vi "SetSequenceNegativeTransitionRegister.vi"(8 "Error In":errorcluster, 10 "Sequence Negative Transition Register":bool[](array[boolean]), 11 "Keithley 7001 In":refnum<visa-resource-name>) -> (0 "Error Out":errorcluster, 3 "Keithley 7001 Out":refnum<visa-resource-name>)   [LabVIEW 2012, in "Keithley-7001.lvlib"]
uses:
  Keithley-7001.lvlib
panel:
  # "Lay1"
  # "Lay2"
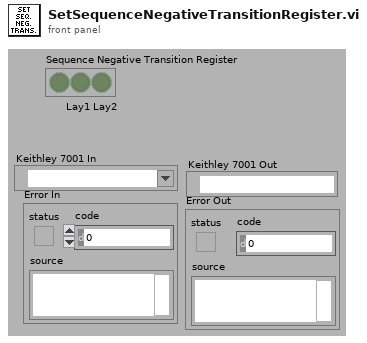
[diagram p1: front panel]
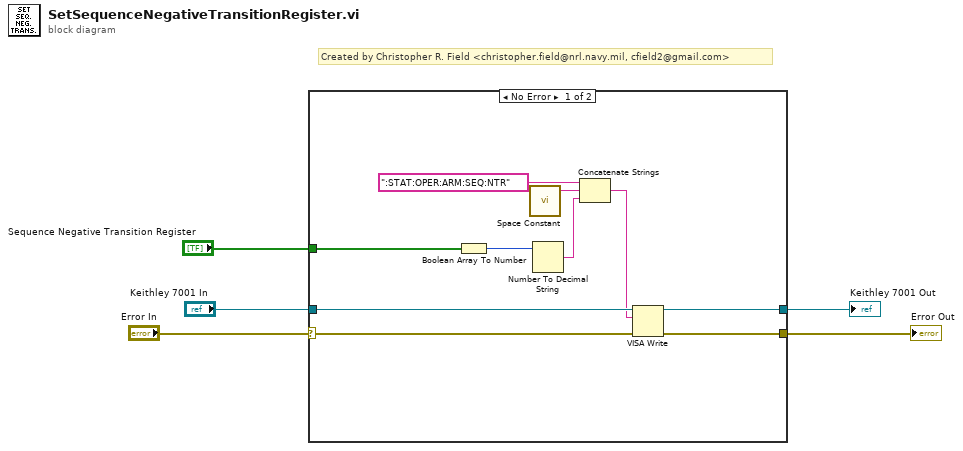
[diagram p0: block diagram]
diagram:
  # "Created by Christopher R. Field <christopher.field@nrl.navy.mil, cfield2@gmail.com>"
  n1 = case shown="No Error" "Error In" {
    selector: "Error In" -> [w6 w16]
    tunnel: "Keithley 7001 In" -> [w15 w17]
    tunnel: "Sequence Negative Transition Register" -> [w12 _]
    tunnel: [w8 w17] -> w3
    tunnel: [w7 w16] -> w2
    frame No Error {
      n2 = Boolean Array To Number(Boolean array=w12) -> (number=w11:u32)
      n3 = call <vilib>:"Space Constant.vi"() -> ("String"=w13:string)
      n4 = Number To Decimal String(number=w11) -> (decimal integer string=w10:string)  [unwired: 1 in]
      n5 = Concatenate Strings(":STAT:OPER:ARM:SEQ:NTR", w13, w10) -> (w9:string)
      n6 = VISA Write(VISA resource name=w15, write buffer=w9, error in (no error)=w6) -> (VISA resource name out=w8:refnum<visa-resource-name>, error out=w7:errorcluster)  [unwired: 1 out]
    }
    frame Error {
    }
  }
  "Keithley 7001 Out" <- w3
  "Error Out" <- w2
